vi "ChartHistoryToXYGraph.vi"(1 "Xo":dbl, 2 "Chart History":dbl[][](array[numeric])) -> (0 "Cap Voltage Graph":cluster{u32[], dbl[]}[](graph))   [LabVIEW 2016]
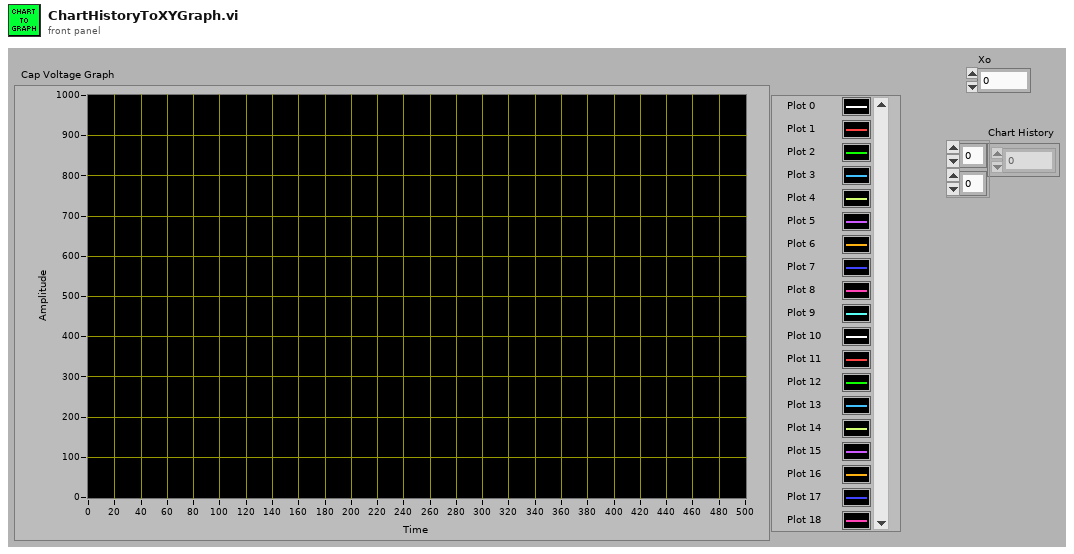
[diagram p1: front panel]
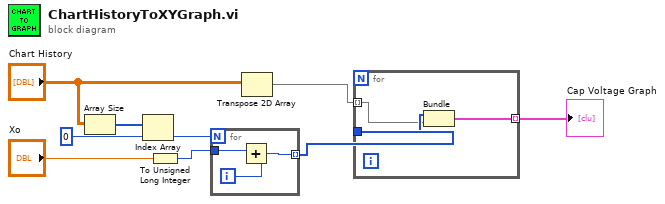
[diagram p0: block diagram]
diagram:
  n1 = Array Size(array="Chart History") -> (size(s)=w3:i32[])
  n2 = Index Array(array=w3, index=0) -> (element=w2:i32)
  n3 = To Unsigned Long Integer(number="Xo") -> (unsigned 32bit integer=w9:u32)
  n4 = for {
    N: w2 -> [_]
    tunnel: w9 -> [w12]
    tunnel: [w10] -> w7 mode=indexing
    i -> [w11]
    n5 = Add(x=w12, y=w11) -> (x+y=w10:u32)
  }
  n6 = Transpose 2D Array(2D array="Chart History") -> (transposed array=w6:dbl[][])
  n7 = for {
    tunnel: w6 -> [w13] mode=indexing
    tunnel: w7 -> [w14]
    tunnel: [w15] -> w8 mode=indexing
    n8 = Bundle(w14, w13) -> (w15:cluster{u32[], dbl[]})  [unwired: 1 in]
  }
  "Cap Voltage Graph" <- w8
